vi "sv_Swept Sine Processor.vi"(6 "RMS level":bool, 8 "error in (no error)":errorcluster, 10 "data to process [V]":cluster{"stimulus":dbl[], "response":dbl[]} {"response" format="%.2f"; "stimulus" format="%.2f"}, 11 "swept sine task in":T2={"source settings"={"AO task name"="", "source"=[]}, "stimulus settings"={"stimulus task name"="", "stimulus"=[]}, "response(s) settings"={"response task name"="", "response"=[]}, "measurement settings"={"AI sampling frequency"=51200.0, "AO sampling frequency"=1024.0, "AI block size"=1024, "AO block Size"=1024, "block duration [ms]"=1024.0, "number of AI channels"=0, "device propagation delay [samples]"=0.0, "total propagation time [samples]"=0.0, "DUT propagation time [ms]"=0.0}, "linlog"=enum."linear", "repeat"=enum."off", "frequency list"=[1.0], "amplitude list"=[1.0], "settling time"={"settle time"=0.015599999576807022, "settle cycles"=5}, "integration time"={"integration time"=0.015599999576807022, "integration cycles"=5}, "frequencies indices"={"AI freq index"=0, "AO freq index"=5}, "read marks"={"write index"=0, "read index"=0, "freq start index"=0, "freq stop index"=0, "# extracted"=0, "buffer type"=enum."Invalid buffer", "read/write indices"=[], "AO index"=0, "AI index"=0, "settled"=FALSE, "integration done"=FALSE}, "harmonic settings"={"maximum THD harmonic"=5, "harmonic mapping"=[1], "units"={"THD unit"=enum."%", "nth harmonic unit"=enum."%", "SINAD unit"=enum."dB", "THD+N unit"=enum."dB"}}, "auto resolution settings"={"auto max step"=512, "slow threshold db"=6.0, "fast threshold db"=1.0}, "auto level settings"={"auto level enable"=FALSE, "auto level channel"=6, "ideal ref"=1.0, "max level"=10.0, "ref upper deviation db"=3.0, "ref lower deviation db"=-3.0}, "offset"=1.0, "ramping rate"=0.0, "phase"=0.0, "initialize"=FALSE} {"phase" format="%.2f"; "response(s) settings"."response"."channel info"."pregain" format="%.2f"; "response(s) settings"."response"."channel info"."weighting filter" items=["Linear", "A-weighting", "B-weighting", "C-weighting", "ITU-R 468-4", "Dolby", "CCITT", "C-message", "Wb", "Wc", "Wd", "We", "Wf", "Wh", "Wj", "Wk", "Wm", "AES17 20 kHz lowpass", "AES17 40 kHz lowpass", "AES17 20 kHz highpass", "AES17 40 kHz highpass"]; "response(s) settings"."response"."channel info"."dB reference" format="%^.1e"; "response(s) settings"."response"."channel info"."engineering units" items=["custom..."=0, "V"=1, "A"=21, "C"=30, "pC"=31, "s"=32, "-"=29, "Pa"=2, "N"=20, "g"=3, "m/s^2"=4, "m/s"=5, "m"=6, "mm/s"=12, "mm"=13, "micron/s"=14, "micron"=15, "in/s^2"=7, "in/s"=8, "in"=9, "mil/s"=10, "mil"=11, "rad/s^2"=16, "rad/s"=17, "rad"=18, "deg/s^2"=26, "deg/s"=27, "deg"=28, "RPM"=22, "cycle/s^2"=23, "Hz"=24, "cycle"=25, "strain"=19]; "response(s) settings"."response"."channel info"."sensor sensitivity" format="%#_5f"; "stimulus settings"."stimulus"."channel info"."pregain" format="%.2f"; "stimulus settings"."stimulus"."channel info"."weighting filter" items=["Linear", "A-weighting", "B-weighting", "C-weighting", "ITU-R 468-4", "Dolby", "CCITT", "C-message", "Wb", "Wc", "Wd", "We", "Wf", "Wh", "Wj", "Wk", "Wm", "AES17 20 kHz lowpass", "AES17 40 kHz lowpass", "AES17 20 kHz highpass", "AES17 40 kHz highpass"]; "stimulus settings"."stimulus"."channel info"."dB reference" format="%^.1e"; "stimulus settings"."stimulus"."channel info"."engineering units" items=["custom..."=0, "V"=1, "A"=21, "C"=30, "pC"=31, "s"=32, "-"=29, "Pa"=2, "N"=20, "g"=3, "m/s^2"=4, "m/s"=5, "m"=6, "mm/s"=12, "mm"=13, "micron/s"=14, "micron"=15, "in/s^2"=7, "in/s"=8, "in"=9, "mil/s"=10, "mil"=11, "rad/s^2"=16, "rad/s"=17, "rad"=18, "deg/s^2"=26, "deg/s"=27, "deg"=28, "RPM"=22, "cycle/s^2"=23, "Hz"=24, "cycle"=25, "strain"=19]; "stimulus settings"."stimulus"."channel info"."sensor sensitivity" format="%#_5f"; "ramping rate" format="%.4f"; "offset" format="%.2f"; "auto level settings"."ref lower deviation db" format="%.4f"; "auto level settings"."ref upper deviation db" format="%.4f"; "auto level settings"."max level" format="%.4f"; "auto level settings"."ideal ref" format="%.4f"; "auto resolution settings"."fast threshold db" format="%.4f"; "auto resolution settings"."slow threshold db" format="%.4f"; "harmonic settings"."maximum THD harmonic" max=10 step=1; "integration time"."integration time" format="%.2p"; "settling time"."settle time" format="%.2p"; "amplitude list" format="%.2f"; "frequency list" format="%.2f"; "measurement settings"."DUT propagation time [ms]" format="%.2f"; "measurement settings"."AO sampling frequency" format="%.2f"; "measurement settings"."AI sampling frequency" format="%.2f"}) -> (0 "error out":errorcluster, 1 "processed frequency (Hz)":dbl format="%.2f", 2 "swept sine measurements":T1 {"scaled response magnitude" format="%.3f"; "Harm[]" format="%.2f"; "THD" format="%.2f"; "Im [response]" format="%.2f"; "Re [response]" format="%.2f"; "Im [stimulus]" format="%.2f"; "Re [stimulus]" format="%.2f"; "RMS response" format="%.2f"; "RMS stimulus" format="%.2f"}, 3 "swept sine task out":T2={"source settings"={"AO task name"="", "source"=[]}, "stimulus settings"={"stimulus task name"="", "stimulus"=[]}, "response(s) settings"={"response task name"="", "response"=[]}, "measurement settings"={"AI sampling frequency"=51200.0, "AO sampling frequency"=1024.0, "AI block size"=1024, "AO block Size"=1024, "block duration [ms]"=1024.0, "number of AI channels"=0, "device propagation delay [samples]"=0.0, "total propagation time [samples]"=0.0, "DUT propagation time [ms]"=0.0}, "linlog"=enum."linear", "repeat"=enum."off", "frequency list"=[1.0], "amplitude list"=[1.0], "settling time"={"settle time"=0.015599999576807022, "settle cycles"=5}, "integration time"={"integration time"=0.015599999576807022, "integration cycles"=5}, "frequencies indices"={"AI freq index"=0, "AO freq index"=5}, "read marks"={"write index"=0, "read index"=0, "freq start index"=0, "freq stop index"=0, "# extracted"=0, "buffer type"=enum."Invalid buffer", "read/write indices"=[], "AO index"=0, "AI index"=0, "settled"=FALSE, "integration done"=FALSE}, "harmonic settings"={"maximum THD harmonic"=5, "harmonic mapping"=[1], "units"={"THD unit"=enum."%", "nth harmonic unit"=enum."%", "SINAD unit"=enum."dB", "THD+N unit"=enum."dB"}}, "auto resolution settings"={"auto max step"=512, "slow threshold db"=6.0, "fast threshold db"=1.0}, "auto level settings"={"auto level enable"=FALSE, "auto level channel"=6, "ideal ref"=1.0, "max level"=10.0, "ref upper deviation db"=3.0, "ref lower deviation db"=-3.0}, "offset"=1.0, "ramping rate"=0.0, "phase"=0.0, "initialize"=FALSE} {"phase" format="%.2f"; "response(s) settings"."response"."channel info"."pregain" format="%.2f"; "response(s) settings"."response"."channel info"."weighting filter" items=["Linear", "A-weighting", "B-weighting", "C-weighting", "ITU-R 468-4", "Dolby", "CCITT", "C-message", "Wb", "Wc", "Wd", "We", "Wf", "Wh", "Wj", "Wk", "Wm", "AES17 20 kHz lowpass", "AES17 40 kHz lowpass", "AES17 20 kHz highpass", "AES17 40 kHz highpass"]; "response(s) settings"."response"."channel info"."dB reference" format="%^.1e"; "response(s) settings"."response"."channel info"."engineering units" items=["custom..."=0, "V"=1, "A"=21, "C"=30, "pC"=31, "s"=32, "-"=29, "Pa"=2, "N"=20, "g"=3, "m/s^2"=4, "m/s"=5, "m"=6, "mm/s"=12, "mm"=13, "micron/s"=14, "micron"=15, "in/s^2"=7, "in/s"=8, "in"=9, "mil/s"=10, "mil"=11, "rad/s^2"=16, "rad/s"=17, "rad"=18, "deg/s^2"=26, "deg/s"=27, "deg"=28, "RPM"=22, "cycle/s^2"=23, "Hz"=24, "cycle"=25, "strain"=19]; "response(s) settings"."response"."channel info"."sensor sensitivity" format="%#_5f"; "stimulus settings"."stimulus"."channel info"."pregain" format="%.2f"; "stimulus settings"."stimulus"."channel info"."weighting filter" items=["Linear", "A-weighting", "B-weighting", "C-weighting", "ITU-R 468-4", "Dolby", "CCITT", "C-message", "Wb", "Wc", "Wd", "We", "Wf", "Wh", "Wj", "Wk", "Wm", "AES17 20 kHz lowpass", "AES17 40 kHz lowpass", "AES17 20 kHz highpass", "AES17 40 kHz highpass"]; "stimulus settings"."stimulus"."channel info"."dB reference" format="%^.1e"; "stimulus settings"."stimulus"."channel info"."engineering units" items=["custom..."=0, "V"=1, "A"=21, "C"=30, "pC"=31, "s"=32, "-"=29, "Pa"=2, "N"=20, "g"=3, "m/s^2"=4, "m/s"=5, "m"=6, "mm/s"=12, "mm"=13, "micron/s"=14, "micron"=15, "in/s^2"=7, "in/s"=8, "in"=9, "mil/s"=10, "mil"=11, "rad/s^2"=16, "rad/s"=17, "rad"=18, "deg/s^2"=26, "deg/s"=27, "deg"=28, "RPM"=22, "cycle/s^2"=23, "Hz"=24, "cycle"=25, "strain"=19]; "stimulus settings"."stimulus"."channel info"."sensor sensitivity" format="%#_5f"; "ramping rate" format="%.4f"; "offset" format="%.2f"; "auto level settings"."ref lower deviation db" format="%.4f"; "auto level settings"."ref upper deviation db" format="%.4f"; "auto level settings"."max level" format="%.4f"; "auto level settings"."ideal ref" format="%.4f"; "auto resolution settings"."fast threshold db" format="%.4f"; "auto resolution settings"."slow threshold db" format="%.4f"; "harmonic settings"."maximum THD harmonic" max=10 step=1; "integration time"."integration time" format="%.2p"; "settling time"."settle time" format="%.2p"; "amplitude list" format="%.2f"; "frequency list" format="%.2f"; "measurement settings"."DUT propagation time [ms]" format="%.2f"; "measurement settings"."AO sampling frequency" format="%.2f"; "measurement settings"."AI sampling frequency" format="%.2f"}, 4 "sweep done":bool, 5 "%done":dbl format="%.2f")   [LabVIEW 2017, in "SoundVib_SweptSine.lvlib"]
uses:
  <vilib>/addons/Sound and Vibration/svt_Swept Sine/SoundVib_SweptSine.lvlib
  <vilib>/addons/Sound and Vibration/svt_Swept Sine/subVIs/sv_Swept Sine Task.ctl
  <vilib>/addons/_NISVFA/_Shared subVIs/Controls/svc_Channel Info.ctl
  <vilib>/addons/_NISVFA/_Shared subVIs/Controls/svc_Engineering Units Text Ring.ctl
  <vilib>/addons/_NISVFA/_Shared subVIs/Controls/svc_Weighting Filter Text Ring.ctl
  <vilib>/addons/Sound and Vibration/svt_Swept Sine/subVIs/sv_Swept Sine Measurements.ctl
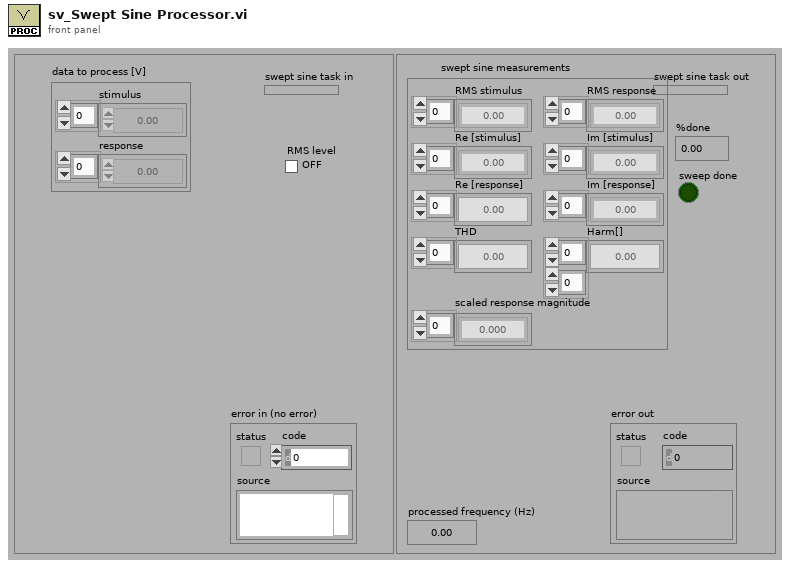
[diagram p1: front panel]
types:
  T1 = typedef "SoundVib_SweptSine.lvlib/sv_Swept Sine Measurements.ctl" = cluster{"RMS stimulus":dbl[], "RMS response":dbl[], "Re [stimulus]":dbl[], "Im [stimulus]":dbl[], "Re [response]":dbl[], "Im [response]":dbl[], "THD":dbl[], "Harm[]":dbl[][], "scaled response magnitude":dbl[]}
  T2 = typedef "SoundVib_SweptSine.lvlib/sv_Swept Sine Task.ctl" = cluster{"source settings":cluster{"AO task name":refnum<k21>, "source":cluster{"AO physical channel":tag}[]}, "stimulus settings":cluster{"stimulus task name":refnum<k21>, "stimulus":cluster{"stimulus physical channel":tag, "channel info":T3}[]}, "response(s) settings":cluster{"response task name":refnum<k21>, "response":cluster{"response physical channel":tag, "channel info":T3}[]}, "measurement settings":cluster{"AI sampling frequency":dbl, "AO sampling frequency":dbl, "AI block size":i32, "AO block Size":i32, "block duration [ms]":dbl, "number of AI channels":i32, "device propagation delay [samples]":dbl, "total propagation time [samples]":dbl, "DUT propagation time [ms]":dbl}, "linlog":enum16{"linear", "log"}, "repeat":enum16{"off", "on"}, "frequency list":dbl[], "amplitude list":dbl[], "settling time":cluster{"settle time":dbl, "settle cycles":i32}, "integration time":cluster{"integration time":dbl, "integration cycles":i32}, "frequencies indices":cluster{"AI freq index":i32, "AO freq index":i32}, "read marks":cluster{"write index":u32, "read index":u32, "freq start index":u32, "freq stop index":u32, "# extracted":u32, "buffer type":enum16{"Invalid buffer", "Intermediate buffer", "Final buffer"}, "read/write indices":cluster{"settle time index":u32, "integration time index":u32}[], "AO index":i32, "AI index":i32, "settled":bool, "integration done":bool}, "harmonic settings":cluster{"maximum THD harmonic":u32, "harmonic mapping":u32[], "units":cluster{"THD unit":enum16{"dB", "%"}, "nth harmonic unit":enum16{"dB", "%"}, "SINAD unit":enum16{"dB", "%"}, "THD+N unit":enum16{"dB", "%"}}}, "auto resolution settings":cluster{"auto max step":i32, "slow threshold db":dbl, "fast threshold db":dbl}, "auto level settings":cluster{"auto level enable":bool, "auto level channel":u8, "ideal ref":sgl, "max level":sgl, "ref upper deviation db":sgl, "ref lower deviation db":sgl}, "offset":dbl, "ramping rate":dbl, "phase":dbl, "initialize":bool}
  T3 = typedef "svc_Channel Info.ctl" = cluster{"sensor sensitivity":dbl, "engineering units":T4, "dB reference":dbl, "custom label":string, "weighting filter":T5, "pregain":dbl}
  T4 = typedef "svc_Engineering Units Text Ring.ctl" = u16
  T5 = typedef "svc_Weighting Filter Text Ring.ctl" = u16
  T6 = enum16{"Invalid buffer", "Intermediate buffer", "Final buffer"}
  T7 = cluster{"settle time index":u32, "integration time index":u32}[]
  T8 = cluster{"stimulus physical channel":tag, "channel info":T3}[]
  T9 = cluster{"response physical channel":tag, "channel info":T3}[]
  T10 = cluster{"RMS stimulus":dbl, "RMS response":dbl, "FRF Measurements":cluster{"Re [stimulus]":dbl, "Im [stimulus]":dbl, "Re [response]":dbl, "Im [response]":dbl}, "THD [ratio]":dbl, "harmonic components [ratio]":dbl[]}
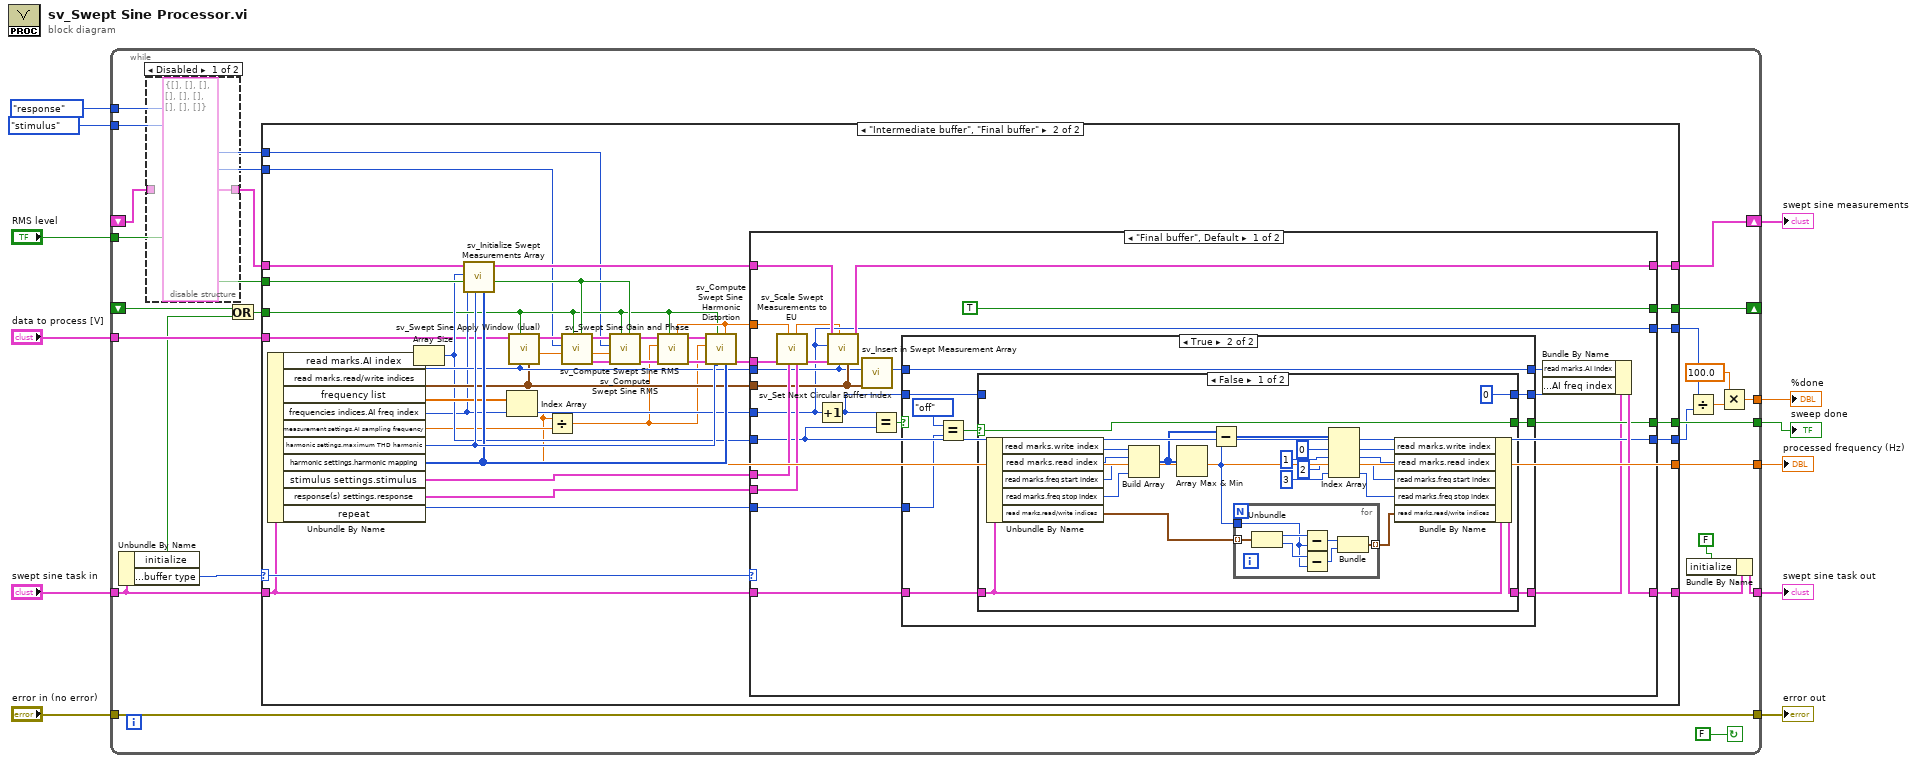
[diagram p0: block diagram]
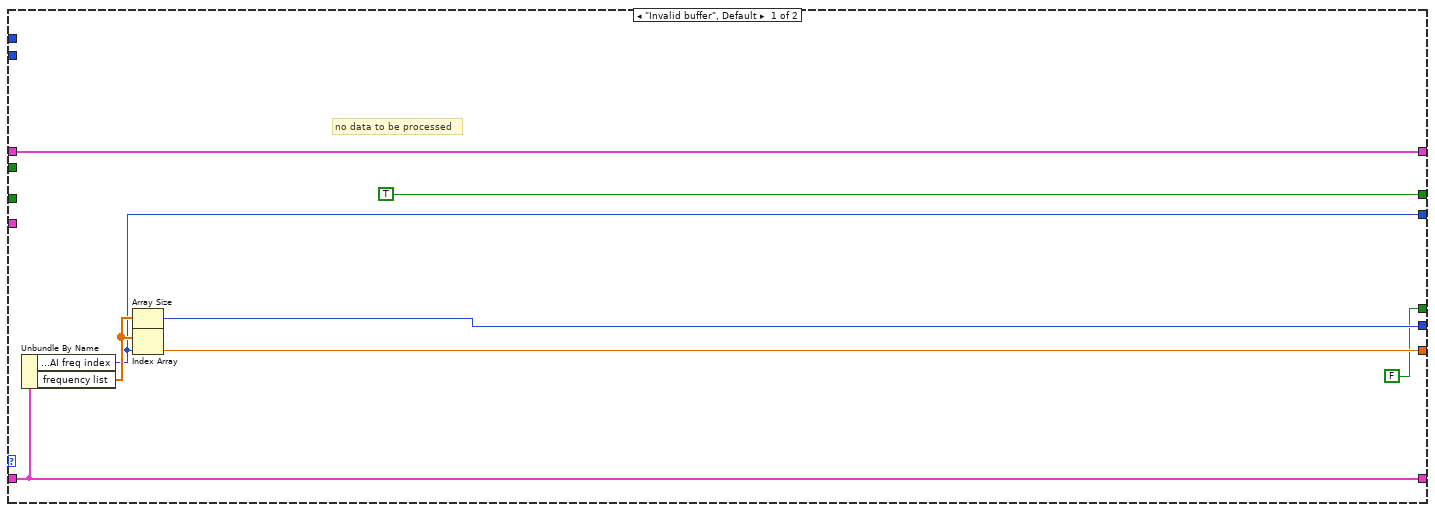
[diagram p3: hidden frame]
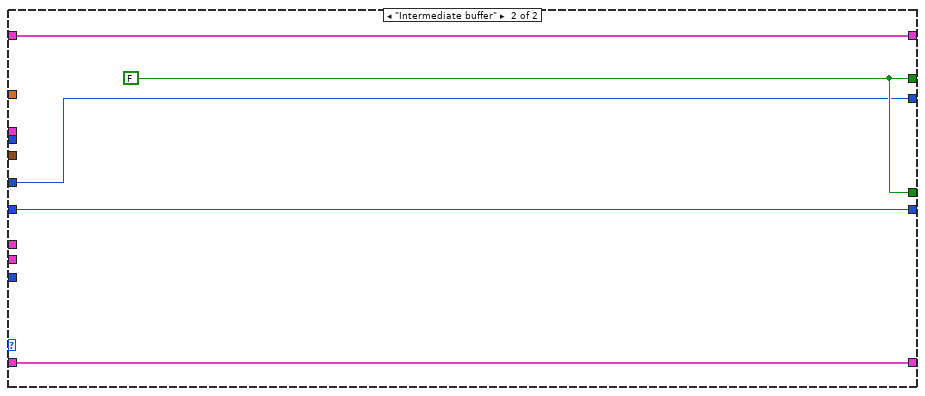
[diagram p6: hidden frame]
diagram:
  n1 = while {
    tunnel: "swept sine task in" -> [w19]
    shift-right: [w36] -> w9
    shift-left: _ -> [w13]
    tunnel: "data to process [V]" -> [w33]
    tunnel: "RMS level" -> [w32]
    shift-right: [w34] -> _
    shift-left: _ -> [w31]
    tunnel: [w16] -> w5
    tunnel: [w21] -> w8
    tunnel: "error in (no error)" -> [w25]
    tunnel: [w25] -> w6
    tunnel: enum16{"stimulus", "response"}."stimulus" ("signal") -> [w29]
    tunnel: enum16{"stimulus", "response"}."response" ("signal") -> [w28]
    tunnel: [w27] -> w2
    tunnel: [w26] -> w1
    stop <- FALSE continue-if-true
    n2 = Unbundle By Name(w19) -> ("initialize"=w18:bool, "read marks.buffer type"=w35:T6)
    n3 = disable-structure shown="Disabled" {
      disable-tunnel: [T1 {"RMS stimulus"=[], "RMS response"=[], "Re [stimulus]"=[], "Im [stimulus]"=[], "Re [response]"=[], "Im [response]"=[], "THD"=[], "Harm[]"=[], "scaled response magnitude"=[]} ("measurements out") w39] -> w14
      disable-tunnel: w13 -> [_ w39]
      frame Disabled {
      }
      frame Enabled {
      }
    }
    n4 = Or(x=w31, y=w18) -> (x .or. y?=w30:bool)
    n5 = case shown="\"Intermediate buffer\", \"Final buffer\"" w35 {
      selector: w35 -> [_ w86]
      tunnel: [w46 w87] -> w36
      tunnel: [TRUE ("reset") w85] -> w34
      tunnel: [w45 w68] -> w17
      tunnel: w19 -> [w45 w75]
      tunnel: w14 -> [w46 w66]
      tunnel: w33 -> [_ w54]
      tunnel: w32 -> [_ w65]
      tunnel: w30 -> [_ w59]
      tunnel: [w44 w61] -> w24
      tunnel: w29 -> [_ w57]
      tunnel: w28 -> [_ w56]
      tunnel: [w42 w51] -> w27
      tunnel: [FALSE w49] -> w26
      tunnel: [w40 w48] -> w20
      frame "Invalid buffer", Default {
        # "no data to be processed"
        n6 = Unbundle By Name(w45) -> ("frequencies indices.AI freq index"=w40:i32, "frequency list"=w43:dbl[])
        n7 = Array Size(array=w43) -> (size(s)=w44:i32)
        n8 = Index Array(array=w43, index=w40) -> (element=w42:dbl)
      }
      frame "Intermediate buffer", "Final buffer" {
        n9 = Unbundle By Name(w75) -> ("read marks.AI index"=w70:i32, "read marks.read/write indices"=w69:T7, "frequency list"=w63:dbl[], "frequencies indices.AI freq index"=w58:i32, "measurement settings.AI sampling frequency"=w52:dbl, "harmonic settings.maximum THD harmonic"=w74:u32, "harmonic settings.harmonic mapping"=w73:u32[], "stimulus settings.stimulus"=w72:T8, "response(s) settings.response"=w71:T9, "repeat"=w62:enum16{"off", "on"})
        n10 = Array Size(array=w63) -> (size(s)=w60:i32)
        n11 = call <vilib>:"sv_Initialize Swept Measurements Array.vi"("harmonic mapping"=w73, "maximum THD harmonic"=w74, "AI freq index"=w58, "RMS level"=w65, "# of points"=w60, "measurements in"=w66) -> ("dup RMS level"=w64:bool, "measurements out"=w67:T1)  [unwired: 4 in]
        n12 = Index Array(array=w63, index=w58) -> (element=w51:dbl)
        n13 = call <vilib>:"sv_Swept Sine Apply Window (dual).vi"("read/write indices"=w69, "AI index"=w70, "reset phase"=w59, "data to process"=w54) -> ("ENBW"=w82:dbl, "windowed data"=w77:cluster{"stimulus":dbl[], "response":dbl[]})  [unwired: 6 in]
        n14 = Divide(x=w51, y=w52) -> (x/y=w50:dbl)
        n15 = call <vilib>:"sv_Compute Swept Sine RMS.vi"("RMS level"=w64, "reset"=w59, "ENBW"=w82, "signal"=w57, "windowed data"=w77) -> ("unscaled measurements out"=w80:T10, "dup ENBW"=w79:dbl, "dup windowed data"=w81:cluster{"stimulus":dbl[], "response":dbl[]})  [unwired: 4 in]
        n16 = call <vilib>:"sv_Compute Swept Sine RMS.vi"("RMS level"=w64, "reset"=w59, "unscaled measurements in"=w80, "ENBW"=w79, "signal"=w56, "windowed data"=w81) -> ("unscaled measurements out"=w84:T10, "dup windowed data"=w76:cluster{"stimulus":dbl[], "response":dbl[]})  [unwired: 3 in, 1 out]
        n17 = call <vilib>:"sv_Swept Sine Gain and Phase.vi"("reset"=w59, "unscaled measurements in"=w84, "frequency [normalized]"=w50, "windowed data"=w76) -> ("unscaled measurements out"=w55:T10, "dup windowed data"=w53:cluster{"stimulus":dbl[], "response":dbl[]}, "unscaled response magnitude"=w78:dbl)  [unwired: 5 in]
        n18 = call <vilib>:"sv_Compute Swept Sine Harmonic Distortion.vi"("harmonic mapping"=w73, "unscaled \nresponse magnitude"=w78, "maximum THD harmonic"=w74, "reset"=w59, "unscaled measurements in"=w55, "frequency (normalized)"=w50, "windowed data"=w53) -> ("unscaled measurements out"=w83:T10)  [unwired: 3 in, 1 out]
        n19 = case shown="\"Final buffer\", Default" w86 {
          tunnel: [w108 w158] -> w87
          tunnel: [TRUE ("reset") w156] -> w85
          tunnel: [w109 w159] -> w68
          tunnel: w83 -> [w106 _]
          tunnel: w78 -> [w89 _]
          tunnel: w75 -> [w94 w159]
          tunnel: w72 -> [w105 _]
          tunnel: w71 -> [w104 _]
          tunnel: w67 -> [w103 w158]
          tunnel: w58 -> [w90 w155]
          tunnel: w70 -> [w101 _]
          tunnel: w69 -> [w102 _]
          tunnel: w62 -> [w98 _]
          tunnel: [w100 w157] -> w61
          tunnel: w60 -> [w100 w157]
          tunnel: [w97 w156] -> w49
          tunnel: [w90 w155] -> w48
          frame "Final buffer", Default {
            n20 = call <vilib>:"sv_Scale Swept Measurements to EU.vi"("response(s) settings.response"=w104, "stimulus settings.stimulus"=w105, "unscaled response magnitude in"=w89, "unscaled measurements"=w106) -> ("scaled measurements"=w107:T10, "unscaled response magnitude out"=w88:dbl)  [unwired: 6 in]
            n21 = Increment(x=w90) -> (x+1=w96:i32)
            n22 = call <vilib>:"sv_Insert in Swept Measurement Array.vi"("read/write indices"=w102, "AI index"=w101, "unscaled response magnitude"=w88, "scaled measurements in"=w107, "AI freq index"=w90, "measurements in"=w103) -> ("measurements out"=w108:T1)  [unwired: 5 in]
            n23 = call <vilib>:"sv_Set Next Circular Buffer Index.vi"("read/write indices"=w102, "current index"=w101) -> ("new index"=w93:i32)  [unwired: 9 in]
            n24 = Equal?(x=w96, y=w100) -> (x = y?=w99:bool)
            n25 = case shown="True" w99 {
              selector: w99 -> [w114 _]
              tunnel: w98 -> [_ w122]
              tunnel: [w114 w115] -> w97
              tunnel: [w113 w120] -> w91
              tunnel: w96 -> [w113 w119]
              tunnel: w94 -> [w112 w118]
              tunnel: [w112 w116] -> w95
              tunnel: w93 -> [w111 w121]
              tunnel: [w111 w121] -> w92
              frame False {
              }
              frame True {
                n26 = Equal?(x=enum16{"off", "on"}."off" ("y"), y=w122) -> (x = y?=w117:bool)
                n27 = case shown="False" w117 {
                  selector: w117 -> [w127 w154]
                  tunnel: [0 ("t") w153] -> w120
                  tunnel: w119 -> [_ w153]
                  tunnel: w118 -> [w130 w152]
                  tunnel: [w128 w152] -> w116
                  tunnel: [w127 w154] -> w115
                  frame False {
                    n28 = Unbundle By Name(w130) -> ("read marks.write index"=w144:u32, "read marks.read index"=w143:u32, "read marks.freq start index"=w142:u32, "read marks.freq stop index"=w141:u32, "read marks.read/write indices"=w126:T7)
                    n29 = Build Array(w144, w143, w142, w141) -> (w140:u32[])
                    n30 = Array Max & Min(array=w140) -> (min value=w125:u32)  [unwired: 3 out]
                    n31 = Subtract(x=w140, y=w125) -> (x-y=w139:u32[])
                    n32 = for {
                      tunnel: w126 -> [w151] mode=indexing
                      tunnel: w125 -> [w148]
                      tunnel: [w145] -> w124 mode=indexing
                      n33 = Unbundle(w151) -> ("settle time index"=w150:u32, "integration time index"=w149:u32)
                      n34 = Subtract(x=w150, y=w148) -> (x-y=w147:u32)
                      n35 = Subtract(x=w149, y=w148) -> (x-y=w146:u32)
                      n36 = Bundle(w147, w146) -> (w145:cluster{u32, u32})  [unwired: 1 in]
                    }
                    n37 = Index Array(array=w139, index #1=0 ("index"), index #2=1 ("index"), index #3=2 ("index"), index #4=3 ("index")) -> (element #1=w134:u32, element #2=w133:u32, element #3=w132:u32, element #4=w131:u32)
                    n38 = Bundle By Name(cluster=w130, "read marks.write index"=w134, "read marks.read index"=w133, "read marks.freq start index"=w132, "read marks.freq stop index"=w131, "read marks.read/write indices"=w124) -> (w128:T2)
                  }
                  frame True {
                  }
                }
              }
            }
            n39 = Bundle By Name(cluster=w95, "read marks.AI index"=w92, "frequencies indices.AI freq index"=w91) -> (w109:T2)
          }
          frame "Intermediate buffer" {
            w156 = FALSE ("reset")
          }
        }
      }
    }
    n40 = Bundle By Name(cluster=w17, "initialize"=FALSE) -> (w16:T2)
    n41 = Divide(x=w20, y=w24) -> (x/y=w22:dbl)
    n42 = Multiply(x=100.0, y=w22) -> (x*y=w21:dbl)
  }
  "error out" <- w6
  "swept sine task out" <- w5
  "sweep done" <- w1
  "swept sine measurements" <- w9
  "%done" <- w8
  "processed frequency (Hz)" <- w2
